vi "Host Main.vi"() -> ()   [LabVIEW 2015, in "SystemLink Tag Module tests.lvlib"]
doc: "This application launches and executes the Tag Bus Data framework configuration for the specified target alias. This is a simple example of the framework API functions, but may also be a suitable starting point for a Host UI or Thick Client that is running a local version of the framework."
uses:
  SystemLink Tag Module tests.lvlib
  <vilib>/NI/Module Execution Interface/Engine Runtime/Execution States.ctl
  <vilib>/NI/Module Execution Interface/Engine Runtime/Fault.ctl
  <vilib>/NI/Tag Bus Module Framework/runtime/error classification.ctl
  <vilib>/NI/Current Value Table/DataTypes/String_Write.vi
  <vilib>/NI/Current Value Table/DataTypes/I32_Write.vi
  <vilib>/NI/Current Value Table/DataTypes/Double_Write.vi
  <vilib>/NI/Current Value Table/DataTypes/String_Read.vi
  <vilib>/NI/Current Value Table/DataTypes/I32_Read.vi
  <vilib>/NI/Current Value Table/DataTypes/Double_Read.vi
  <vilib>/NI/Current Value Table/Type to Enum.vi
  <vilib>/NI/Current Value Table/DataTypes/String_Type To Enum.vi
  <vilib>/NI/Current Value Table/DataTypes/I32_Type To Enum.vi
  <vilib>/NI/Current Value Table/DataTypes/Double_Type To Enum.vi
  <vilib>/NI/Current Value Table/FGVs/CVT Globals.vi
  <vilib>/NI/Current Value Table/FGVs/Tag Memory.vi
  <vilib>/NI/Current Value Table/Memory Block.vi
  <vilib>/NI/Current Value Table/DataTypes/String_Memory Block.vi
  <vilib>/NI/Current Value Table/DataTypes/I32_Memory Block.vi
  <vilib>/NI/Current Value Table/DataTypes/Double_Memory Block.vi
  <vilib>/NI/Module Execution Interface/Engine Runtime/Engine Runtime Interface.lvclass
  <vilib>/NI/DCAF/Tag Editor Core/Framework Configuration Classes/target runtime/PL_Target Runtime.lvclass
  <vilib>/NI/Current Value Table/Current Value Table.lvlib
  <vilib>/NI/Tag Bus Module Framework/runtime/TBM module execution interface.lvclass
panel:
  in  "Double In":dbl
  in  "I32 In":i32
  in  "Strin In":string
  out "Double Out":dbl
  out "I32 Out":i32
  out "String Out":string
  in  "configuration file path":path=path "C:/Git/SystemLinkTagModule/Source/testing/SysLink.pcfg"
  in  "target alias":string="PC"
  out "engine status":T4(array[cluster])
  in  "stop":bool
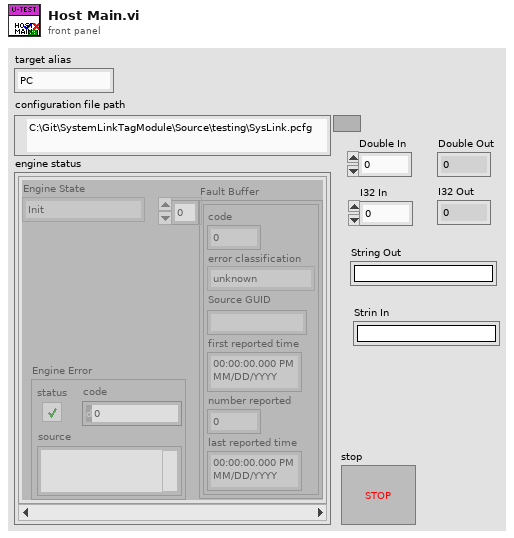
[diagram p1: front panel]
types:
  T1 = typedef "Engine Runtime Interface.lvclass/Execution States.ctl" = enum16{"Init", "Pre-Operational", "Safe-Operational", "Operational", "Stopped"}
  T2 = typedef "Engine Runtime Interface.lvclass/Fault.ctl" = cluster{"code":i32, "error classification":T3, "Source GUID":string, "first reported time":timestamp, "number reported":u32, "last reported time":timestamp}
  T3 = typedef "TBM module execution interface.lvclass/error classification.ctl" = enum16{"unknown", "none", "trivial", "recoverable", "critical"}
  T4 = cluster{"Engine State":T1, "Fault Buffer":T2[], "Engine Error":errorcluster}[]
  T5 = cluster{"Engine State":T1, "faults":T2[], "Engine Error":errorcluster}
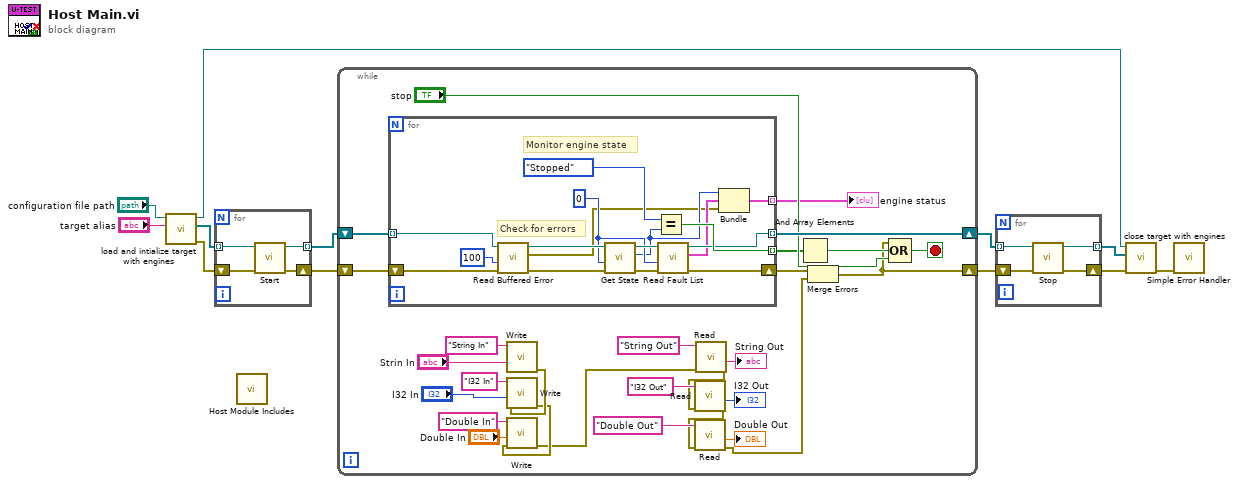
[diagram p0: block diagram]
diagram:
  n1 = call <vilib>:"load and intialize target with engines.vi"("target alias"="target alias", "file path"="configuration file path") -> ("error out"=w9:errorcluster, "engine runtime interfaces"=w8:refnum<class "Engine Runtime Interface.lvclass">[], "target runtime"=w5:refnum<class "PL_Target Runtime.lvclass">)  [unwired: 7 in]
  n2 = for {
    tunnel: [w16] -> w12 mode=indexing
    tunnel: w8 -> [w13] mode=indexing
    shift-right: [w15] -> w2
    shift-left: w9 -> [w14]
    n3 = call-dynamic "Start.vi"("error in"=w14, "Engine Runtime Interface in"=w13) -> ("error out"=w15:errorcluster, "Engine Runtime Interface out"=w16:refnum<class "Engine Runtime Interface.lvclass">)  [unwired: 8 in]
  }
  n4 = call "Host Module Includes.vi"() -> ()  [unwired: 12 in]
  n5 = while {
    shift-right: [w42] -> w11
    shift-left: w12 -> [w44]
    shift-right: [w18] -> w10
    shift-left: w2 -> [w43]
    stop <- w40 stop-if-true
    n6 = for {
      tunnel: w44 -> [w60] mode=indexing
      tunnel: [w51] -> w42 mode=indexing
      tunnel: [w55] -> w37 mode=indexing
      shift-right: [w50] -> w39
      shift-left: w43 -> [w59]
      tunnel: [w45] -> w38 mode=indexing
      w49 = 0 ("timeout (-1)")
      # "Monitor engine state"
      # "Check for errors"
      n7 = call-dynamic "Read Buffered Error.vi"("error in"=w59, "timeout in ms (0)"=100, "Engine Runtime Interface in"=w60) -> ("error out"=w57:errorcluster, "Engine Error"=w46:errorcluster, "Engine Runtime Interface out"=w58:refnum<class "Engine Runtime Interface.lvclass">)  [unwired: 6 in]
      n8 = call-dynamic "Get State.vi"("error in"=w57, "timeout (-1)"=w49, "Engine Runtime Interface in"=w58) -> ("error out"=w53:errorcluster, "Engine State"=w48:T1, "Engine Runtime Interface out"=w52:refnum<class "Engine Runtime Interface.lvclass">)  [unwired: 6 in]
      n9 = Equal?(x=Execution_States."Stopped" ("Engine State"), y=w48) -> (x = y?=w55:bool)
      n10 = call-dynamic "Read Fault List.vi"("error in"=w53, "timeout (-1)"=w49, "Engine Runtime Interface in"=w52) -> ("error out"=w50:errorcluster, "faults"=w47:T2[], "Engine Runtime Interface out"=w51:refnum<class "Engine Runtime Interface.lvclass">)  [unwired: 6 in]
      n11 = Bundle("Engine State"=w48, "faults"=w47, "Engine Error"=w46) -> (w45:T5)  [unwired: 1 in]
    }
    "engine status" <- w38
    n12 = call-poly <vilib>:"Write.vi"("Value"="Strin In", "Tag Name"="String In") -> ("error out"=w23:errorcluster)  [unwired: 9 in]
    n13 = call-poly <vilib>:"Write.vi"("error in (no error)"=w23, "Value"="I32 In", "Tag Name"="I32 In") -> ("error out"=w22:errorcluster)  [unwired: 8 in]
    n14 = call-poly <vilib>:"Write.vi"("error in (no error)"=w22, "Value"="Double In", "Tag Name"="Double In") -> ("error out"=w21:errorcluster)  [unwired: 8 in]
    n15 = call-poly <vilib>:"Read.vi"("error in (no error)"=w21, "Tag Name"="String Out") -> ("error out"=w20:errorcluster, "Value"=→"String Out":string)  [unwired: 8 in]
    n16 = call-poly <vilib>:"Read.vi"("error in (no error)"=w20, "Tag Name"="I32 Out") -> ("error out"=w19:errorcluster, "Value"=→"I32 Out":i32)  [unwired: 8 in]
    n17 = call-poly <vilib>:"Read.vi"("error in (no error)"=w19, "Tag Name"="Double Out") -> ("error out"=w17:errorcluster, "Value"=→"Double Out":dbl)  [unwired: 8 in]
    n18 = And Array Elements(Boolean array=w37) -> (logical AND=w36:bool)
    n19 = Merge Errors(w39, w17) -> (w18:errorcluster)
    n20 = Compound Arithmetic op=OR(w18, w36, "stop") -> (w40:bool)
  }
  n21 = for {
    tunnel: w11 -> [w64] mode=indexing
    shift-right: [w61] -> w4
    shift-left: w10 -> [w63]
    tunnel: [w62] -> w6 mode=indexing
    n22 = call-dynamic "Stop.vi"("error in"=w63, "Engine Runtime Interface in"=w64) -> ("error out"=w61:errorcluster, "Engine Runtime Interface out"=w62:refnum<class "Engine Runtime Interface.lvclass">)  [unwired: 8 in]
  }
  n23 = call <vilib>:"close target with engines.vi"("error in"=w4, "Engine Runtime Interfaces"=w6, "Target Runtime"=w5) -> ("error out"=w1:errorcluster)  [unwired: 8 in]
  n24 = call <vilib>:"Simple Error Handler.vi"("error in (no error)"=w1) -> ()  [unwired: 4 in, 5 out]
